vi "WriteIOValues b2g1.vi"(2 "error in":errorcluster, 3 "Output - Cluster b2g1":T1 {"TS-6 [°C]" format="%.0g"; "TS-5 [°C]" format="%#.2g"; "pHS-1 [pH]" format="%.2g"; "TS-4 [°C]" format="%#.2g"; "FS-2 [l]" format="%.2g"; "FS-1 [l]" format="%.2g"; "DS-1 [bar]" format="%#.2g"; "DFS-1 [l/min]" format="%#.2g"; "FS-3 [l]" format="%.2g"; "DFS-1 [dl]" format="%.0g"}, 4 "input cluster":T2 {"P-5 AUS [min]" max=100 step=1 format="%#_3g"; "P-5 EIN [min]" step=1 format="%#_3g"; "Hysterese [°C]" format="%.1g"; "Dosiergeschw. [l/min]" format="%.2g"; "Dosiermenge [l]" format="%.2g"; "Temp Soll [°C]" format="%.2g"; "Druck Soll [bar]" format="%.2g"; "Füllstand Soll [l]" format="%_3g"; "P-5 Drehzahl [%]" max=100 step=1 format="%#_3g"; "P-4 Drehzahl [%]" max=100 step=1 format="%#_3g"; "V-15 [%]" max=100 step=1 format="%_1g"; "V-13 [%]" max=100 step=1 format="%_1g"}) -> (0 "error out":errorcluster, 1 "output cluster":T1 {"TS-6 [°C]" format="%.0g"; "TS-5 [°C]" format="%#.2g"; "pHS-1 [pH]" format="%.2g"; "TS-4 [°C]" format="%#.2g"; "FS-2 [l]" format="%.2g"; "FS-1 [l]" format="%.2g"; "DS-1 [bar]" format="%#.2g"; "DFS-1 [l/min]" format="%#.2g"; "FS-3 [l]" format="%.2g"; "DFS-1 [dl]" format="%.0g"})   [LabVIEW 2011]
uses:
  Input - Cluster b2g1.ctl
  Output - Cluster b2g1.ctl
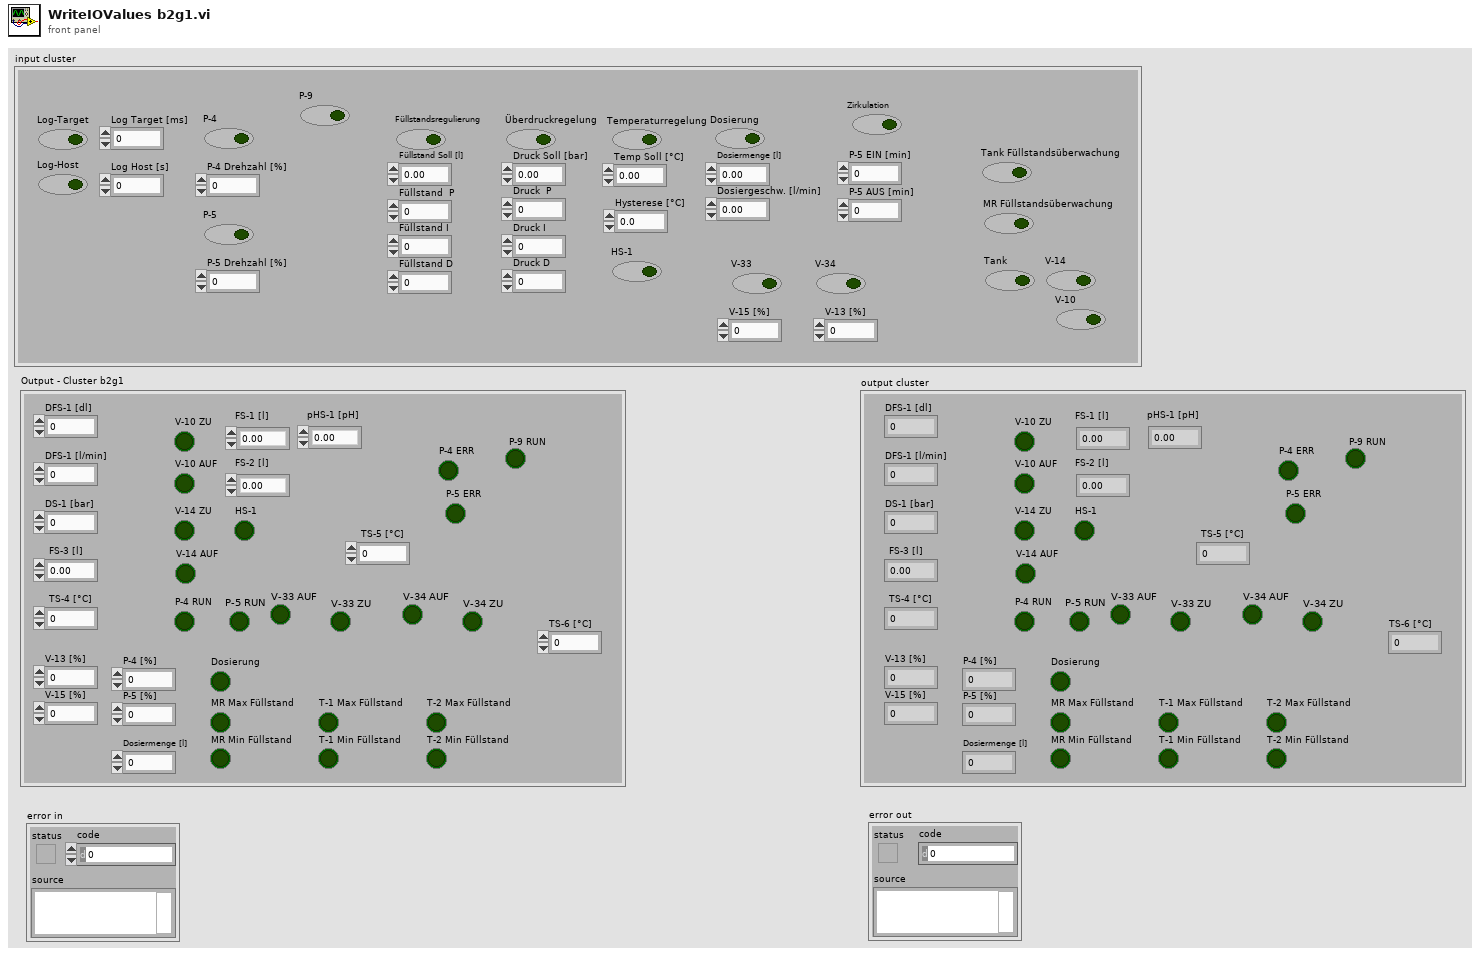
[diagram p1: front panel]
types:
  T1 = typedef "Output - Cluster b2g1.ctl" = cluster{"DFS-1 [dl]":u64, "FS-3 [l]":dbl, "DFS-1 [l/min]":dbl, "DS-1 [bar]":dbl, "V-10 ZU":bool, "V-14 ZU":bool, "FS-1 [l]":dbl, "FS-2 [l]":dbl, "TS-4 [°C]":dbl, "HS-1":bool, "V-13 [%]":u8, "V-15 [%]":u8, "P-4 [%]":u8, "P-5 [%]":u8, "Dosierung":bool, "MR Max Füllstand":bool, "MR Min Füllstand":bool, "Dosiermenge [l]":sgl, "V-14 AUF":bool, "V-10 AUF":bool, "T-1 Max Füllstand":bool, "T-1 Min Füllstand":bool, "T-2 Max Füllstand":bool, "T-2 Min Füllstand":bool, "pHS-1 [pH]":dbl, "P-4 RUN":bool, "P-5 RUN ":bool, "V-33 AUF":bool, "V-33 ZU":bool, "V-34 AUF":bool, "V-34 ZU":bool, "P-4 ERR":bool, "P-5 ERR":bool, "TS-5 [°C]":dbl, "TS-6 [°C]":dbl, "P-9 RUN":bool}
  T2 = typedef "Input - Cluster b2g1.ctl" = cluster{"V-13 [%]":u8, "V-15 [%]":u8, "Log-Target":bool, "P-4":bool, "P-4 Drehzahl [%]":u8, "Temperaturregelung":bool, "Überdruckregelung":bool, "Füllstandsregulierung":bool, "V-10":bool, "Log-Host":bool, "V-14":bool, "P-5":bool, "P-5 Drehzahl [%]":u8, "HS-1":bool, "Füllstand  P":sgl, "Füllstand I":sgl, "Füllstand D":sgl, "Füllstand Soll [l]":sgl, "Druck  P":sgl, "Druck I":sgl, "Druck D":sgl, "Druck Soll [bar]":sgl, "Temp Soll [°C]":sgl, "Dosierung":bool, "Dosiermenge [l]":sgl, "Dosiergeschw. [l/min]":sgl, "Tank":bool, "Hysterese [°C]":sgl, "MR Füllstandsüberwachung":bool, "Tank Füllstandsüberwachung":bool, "Log Target [ms]":u32, "Log Host [s]":u32, "P-5 EIN [min]":u8, "P-5 AUS [min]":u8, "Zirkulation":bool, "V-33":bool, "V-34":bool, "P-9":bool}
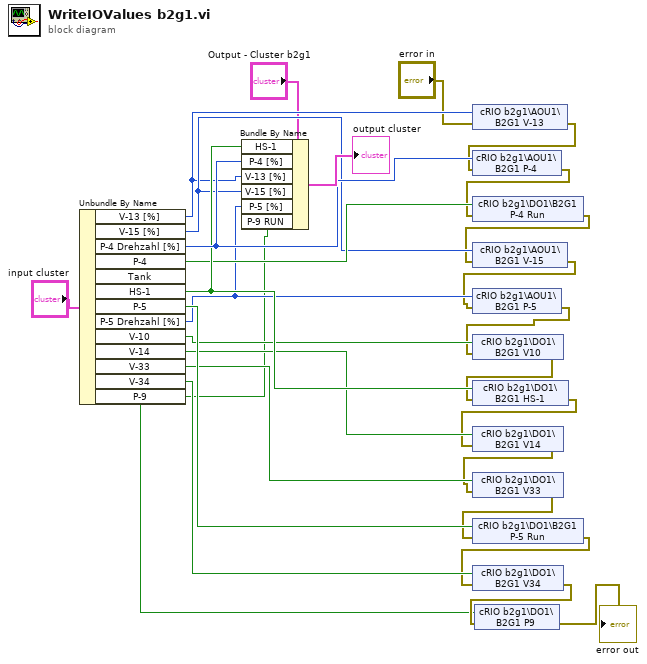
[diagram p0: block diagram]
diagram:
  n1 = Unbundle By Name("input cluster") -> ("V-13 [%]"=w20:u8, "V-15 [%]"=w23:u8, "P-4 Drehzahl [%]"=w27:u8, "P-4"=w25:bool, "HS-1"=w26:bool, "P-5"=w24:bool, "P-5 Drehzahl [%]"=w17:u8, "V-10"=w22:bool, "V-14"=w21:bool, "V-33"=w19:bool, "V-34"=w18:bool, "P-9"=w1:bool)  [unwired: 1 out]
  n2 = Bundle By Name(cluster="Output - Cluster b2g1", "HS-1"=w26, "P-4 [%]"=w27, "V-13 [%]"=w20, "V-15 [%]"=w23, "P-5 [%]"=w17, "P-9 RUN"=w1) -> (→"output cluster":T1)
  n3 = shared-variable "cRIO b2g1\\AOU1\\B2G1 V-13"(w20, error in="error in") -> (error out=w13:errorcluster)
  n4 = shared-variable "cRIO b2g1\\AOU1\\B2G1 P-4"(w27, error in=w13) -> (error out=w12:errorcluster)
  n5 = shared-variable "cRIO b2g1\\DO1\\B2G1 P-4 Run"(w25, error in=w12) -> (error out=w11:errorcluster)
  n6 = shared-variable "cRIO b2g1\\AOU1\\B2G1 V-15"(w23, error in=w11) -> (error out=w10:errorcluster)
  n7 = shared-variable "cRIO b2g1\\AOU1\\B2G1 P-5"(w17, error in=w10) -> (error out=w9:errorcluster)
  n8 = shared-variable "cRIO b2g1\\DO1\\B2G1 V10"(w22, error in=w9) -> (error out=w8:errorcluster)
  n9 = shared-variable "cRIO b2g1\\DO1\\B2G1 HS-1"(w26, error in=w8) -> (error out=w7:errorcluster)
  n10 = shared-variable "cRIO b2g1\\DO1\\B2G1 V14"(w21, error in=w7) -> (error out=w6:errorcluster)
  n11 = shared-variable "cRIO b2g1\\DO1\\B2G1 V33"(w19, error in=w6) -> (error out=w5:errorcluster)
  n12 = shared-variable "cRIO b2g1\\DO1\\B2G1 P-5 Run"(w24, error in=w5) -> (error out=w4:errorcluster)
  n13 = shared-variable "cRIO b2g1\\DO1\\B2G1 V34"(w18, error in=w4) -> (error out=w2:errorcluster)
  n14 = shared-variable "cRIO b2g1\\DO1\\B2G1 P9"(w1, error in=w2) -> (error out=→"error out":errorcluster)
